vi "AfterPage2_UI.vi"(10 "MetaDataObj":refnum<class "MetaDataObj.lvclass">) -> ()   [LabVIEW 2021, in "CIF_Plugin_Generator.lvclass"]
uses:
  CIF_Plugin_Generator.lvclass
  <resource>/dialog/NewProjectWizard/MetaDataObj/MetaDataObj.lvclass
  C:/Program Files/National Instruments/LabVIEW 2021/resource/dialog/NewProjectWizard/MetaDataObj/MetaDataObj.lvclass
  <resource>/dialog/NewProjectWizard/MetaDataObj/MetaDataObj.lvclass/MetaDataObj.ctl
  CIF_Plugin_Generator.lvclass/CIF_Plugin_Generator.ctl
  2b3e1c27-d443-4546-a5b6-192e9e090b09.vi
  <resource>/dialog/NewProjectWizard/MetaDataObj/Accessors/Read Project Root.vi
  <resource>/dialog/NewProjectWizard/MetaDataObj/Accessors/Read Project Name.vi
  <resource>/dialog/NewProjectWizard/MetaDataObj/Accessors/Read Overlay Pixmap.vi
  <vilib>/LabVIEW Icon API/lv_icon/Classes/Icon/Icon.lvclass
  Plugin Generator.lvlib
  <vilib>/CIF Foundation/CIF Utilities/Errors/Errors_CIF_U.lvlib
panel:
  out "To display":string
  out "Plugin Generation Status":string
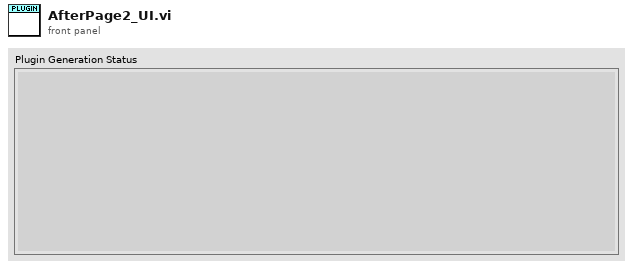
[diagram p1: front panel]
types:
  T1 = typedef "ChannelRegistrar.lvlib/Channel Definition for Scripting.ctl" = cluster{"Name":string, "Direction":T2, "Type":T3}
  T2 = typedef "CIFChannels.lvclass/Direction.ctl" = enum16{"Publisher", "Subscriber"}
  T3 = typedef "ChannelRegistrar.lvlib/Registered Channel Types.ctl" = enum16{"Custom", "Double_Tag", "I64_Tag", "U64_Tag", "U8_FIFO", "CAN_FIFO", "L2Enet_FIFO", "DAQ_FIFO", "Universal_FIFO", "String_Tag"}
  T4 = typedef "Plugin Generator.lvlib/Proto Names.ctl" = cluster{"PascalCase":string, "snake_case":string}
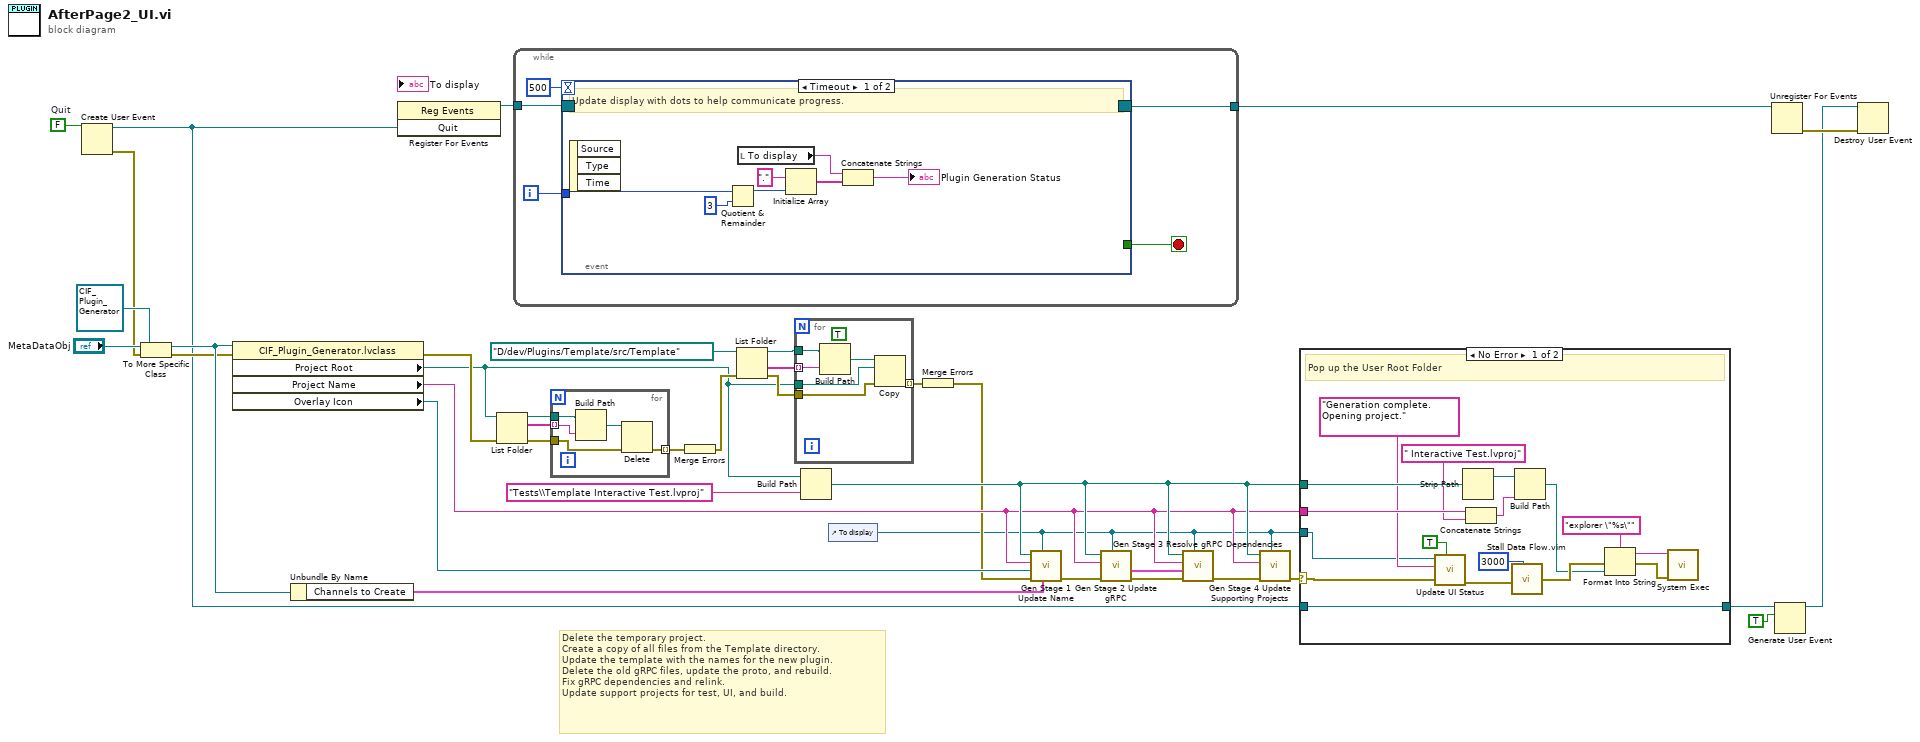
[diagram p0: block diagram]
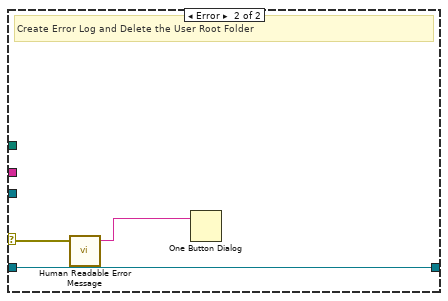
[diagram p2: hidden frame]
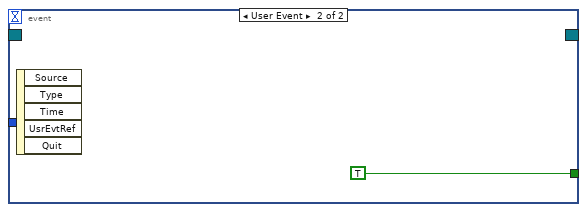
[diagram p3: hidden frame]
diagram:
  w19 = FALSE  # Quit
  # "Delete the temporary project.\nCreate a copy of all files from the Template directory.\nUpdate the template with the names for the new plugin.\nDelete the old gRPC files, update the proto, and rebuild.\nFix gRPC dependencies and relink.\nUpdate support projects for test, UI, and build."
  n1 = Create User Event(user event datatype=w19) -> (user event=w12:refnum<user-event>, error out=w11:errorcluster)  [unwired: 1 in]
  n2 = To More Specific Class(target class=refnum<class "CIF_Plugin_Generator.lvclass"> refnum ("Plugin_Generator.lvclass"), reference="MetaDataObj", error in=w11) -> (specific class reference=w36:refnum<class "CIF_Plugin_Generator.lvclass">, error out=w35:errorcluster)
  n3 = property class="CIF_Plugin_Generator.lvclass"(reference=w36, error in=w35) -> (error out=w30:errorcluster, "Project Root"=w23:path, "Project Name"=w6:string, "Overlay Icon"=w21:refnum<class "Icon.lvclass">)  [unwired: 1 out]
  n4 = Unbundle By Name(w36) -> ("Channels to Create"=w20:T1[])
  n5 = register-events(w12) -> (reference out=w18:refnum<event-registration>)  [unwired: 2 in, 1 out]
  n6 = List Folder(path=w23, error in=w30) -> (path out=w33:path, filenames=w32:string[], error out=w31:errorcluster)  [unwired: 2 in, 1 out]
  n7 = while {
    tunnel: w18 -> [w41]
    tunnel: [w38] -> w16
    i -> [w39]
    stop <- w40 stop-if-true
    n8 = event shown="[0] Timeout" {
      selector: w41 -> [_ _]
      dyn-events: [_ _] -> w38
      timeout: 500 -> [_ _]
      tunnel: [_ TRUE] -> w40
      tunnel: w39 -> [w49 _]
      event Timeout {
        # "Update display with dots to help communicate progress."
        n9 = event-data() -> ()  [unwired: 1 in, 3 out]
        n10 = Quotient & Remainder(x=w49, y=3) -> (x-y*floor(x/y)=w47:i32)  [unwired: 1 out]
        n11 = local read "To display"() -> (w48:string)
        n12 = Initialize Array(".", w47) -> (w45:string[])
        n13 = Concatenate Strings(w48, w45) -> (→"Plugin Generation Status":string)
      }
      event User Event {
        n14 = event-data() -> ()  [unwired: 1 in, 5 out]
      }
    }
  }
  n15 = for {
    tunnel: w33 -> [w55]
    tunnel: w32 -> [w54] mode=indexing
    tunnel: w31 -> [w52]
    tunnel: [w51] -> w29 mode=indexing
    n16 = Build Path(base path=w55, name or relative path=w54) -> (appended path=w53:path)
    n17 = Delete(path (use dialog)=w53, error in=w52) -> (error out=w51:errorcluster)  [unwired: 3 in, 2 out]
  }
  n18 = Merge Errors(w29) -> (w25:errorcluster)
  n19 = List Folder(path=path "D:/dev/Plugins/Template/src/Template" ("source path"), error in=w25) -> (path out=w27:path, folder names=w26:string[], error out=w24:errorcluster)  [unwired: 2 in, 1 out]
  n20 = for {
    tunnel: w27 -> [w61]
    tunnel: w24 -> [w59]
    tunnel: w26 -> [w60] mode=indexing
    tunnel: w23 -> [w57]
    tunnel: [w56] -> w9 mode=indexing
    (unwired) TRUE ("entire hierarchy (F)")
    n21 = Build Path(base path=w61, name or relative path=w60) -> (appended path=w58:path)
    n22 = Copy(8:w59, 10:w57, 11:w58) -> (0:w56:errorcluster)  [unwired: 2 in, 2 out]
  }
  n23 = Build Path(base path=w23, name or relative path="Tests\\Template Interactive Test.lvproj") -> (appended path=w7:path)
  n24 = control-ref of="To display"() -> (w1:refnum<vi>)
  n25 = Merge Errors(w9) -> (w5:errorcluster)
  n26 = call "Gen Stage 1 Update Name.vi"("Channels to Create"=w20, "Staus"=w1, "error in"=w5, "Overlay Icon"=w21, "New Subname"=w6, "Template Project Path"=w7) -> ("error out"=w4:errorcluster)  [unwired: 5 in]
  n27 = call "Gen Stage 2 Update gRPC.vi"("Staus"=w1, "error in"=w4, "New Subname"=w6, "Template Project Path"=w7) -> ("error out"=w3:errorcluster, "Proto Names"=w8:T4)  [unwired: 6 in]
  n28 = call "Gen Stage 3 Resolve gRPC Dependencies.vi"("Staus"=w1, "error in"=w3, "Proto Names"=w8, "New Subname"=w6, "Template Project Path"=w7) -> ("error out"=w2:errorcluster)  [unwired: 6 in]
  n29 = call "Gen Stage 4 Update Supporting Projects.vi"("Staus"=w1, "error in (no error)"=w2, "New Name"=w6, "Template Project Path"=w7) -> ("error out"=w10:errorcluster)  [unwired: 7 in]
  n30 = case shown="No Error" w10 {
    selector: w10 -> [w63 w80]
    tunnel: [w75 w81] -> w13
    tunnel: w12 -> [w75 w81]
    tunnel: w7 -> [w72 _]
    tunnel: w6 -> [w68 _]
    tunnel: w1 -> [w64 _]
    frame No Error {
      # "Pop up the User Root Folder"
      n31 = call "Update UI Status.vi"("Previous Complete"=TRUE, "error in"=w63, "Status to Display"="Generation complete.  Opening project." ("To display"), "String in"=w64) -> ("error out"=w62:errorcluster)  [unwired: 7 in]
      n32 = Strip Path(path=w72) -> (stripped path=w71:path)  [unwired: 1 out]
      n33 = Concatenate Strings(w68, " Interactive Test.lvproj" ("string")) -> (w69:string)
      n34 = call "Stall Data Flow.vim"("value in"=w62, "milliseconds to wait"=u32 3000) -> ("value out"=w74:errorcluster)  [unwired: 1 out]
      n35 = Build Path(base path=w71, name or relative path=w69) -> (appended path=w70:path)
      n36 = Format Into String(format string="explorer \"%s\"", error in=w74, w70) -> (resulting string=w78:string, error out=w76:errorcluster)  [unwired: 1 in]
      n37 = call <vilib>:"System Exec.vi"("error in (no error)"=w76, "command line"=w78) -> ()  [unwired: 6 in, 4 out]
    }
    frame Error {
      # "Create Error Log and Delete the User Root Folder"
      n38 = call <vilib>:"Human Readable Error Message.vi"("error in (no error)"=w80) -> ("Human readable error message"=w79:string)  [unwired: 4 in]
      n39 = One Button Dialog(message=w79) -> ()  [unwired: 1 in, 1 out]
    }
  }
  n40 = Unregister For Events(event registration refnum=w16) -> (error out=w15:errorcluster)  [unwired: 1 in]
  n41 = Generate User Event(user event=w13, event data cluster=TRUE ("event data")) -> (user event out=w14:refnum<user-event>)  [unwired: 2 in, 1 out]
  n42 = Destroy User Event(user event=w14, error in=w15) -> ()  [unwired: 1 out]
